vi "_Get Startup File.vi"(1 "FileName":string="Config") -> (0 "FilePath":path)   [LabVIEW 2015]
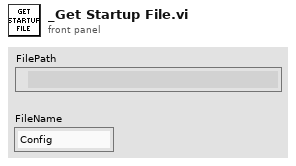
[diagram p1: front panel]
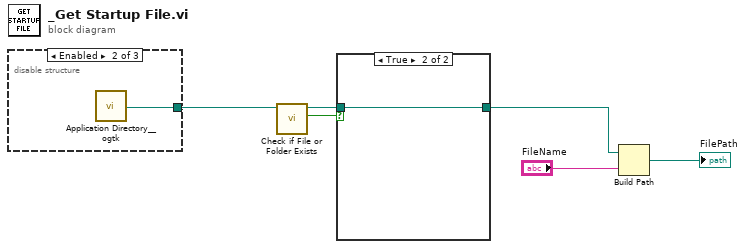
[diagram p0: block diagram]
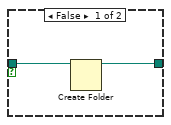
[diagram p2: hidden frame]
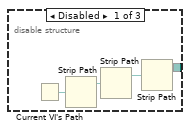
[diagram p3: hidden frame]
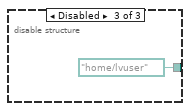
[diagram p4: hidden frame]
diagram:
  n1 = disable-structure shown="Enabled" {
    disable-tunnel: [w7 w11 path "/home/lvuser" ("stripped path")] -> w3
    frame Disabled {
      n2 = Current VI's Path() -> (path=w8:path)
      n3 = Strip Path(path=w8) -> (stripped path=w9:path)  [unwired: 1 out]
      n4 = Strip Path(path=w9) -> (stripped path=w10:path)  [unwired: 1 out]
      n5 = Strip Path(path=w10) -> (stripped path=w7:path)  [unwired: 1 out]
    }
    frame Enabled {
      n6 = call <userlib>:"Application Directory__ogtk.vi"() -> ("Application Directory (+ Relative)"=w11:path)  [unwired: 1 in]
    }
    frame Disabled {
    }
  }
  n7 = call <vilib>:"Check if File or Folder Exists.vi"("path"=w3) -> ("file or folder exists?"=w5:bool, "dup path"=w4:path)  [unwired: 8 in, 1 out]
  n8 = case shown="True" w5 {
    tunnel: w4 -> [w14 w15]
    tunnel: [w13 w15] -> w2
    frame False {
      n9 = Create Folder(path (use dialog)=w14) -> (created path=w13:path)  [unwired: 2 in, 2 out]
    }
    frame True {
    }
  }
  n10 = Build Path(base path=w2, name or relative path="FileName") -> (appended path=→"FilePath":path)
